vi "Configure Signal Track Enabled.vi"(8 "error in (no error)":errorcluster {"code" format="%.0x"}, 9 "signal track enabled (Off)":bool, 11 "instrument handle":refnum<k15>) -> (0 "error out":errorcluster {"code" format="%.0x"}, 3 "instrument handle out":refnum<k15>)   [LabVIEW 2009, in "Keysight XSAn.lvlib"]
doc: "This VI enables or disables signal-tracking.\n\nSupported Models: M9290A, N8973B, N8974B, N8975B, N8976B, N9000A, N9000B, N9010A, N9010B, N9020A, N9020B, N9030A, N9030B, N9038A, N9040B, N9041B, SPN9003A, SPN9026A"
uses:
  <instrlib>/Keysight XSAn/Keysight XSAn.lvlib
  AgXSAn.dll
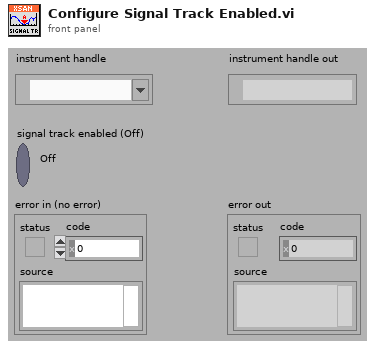
[diagram p1: front panel]
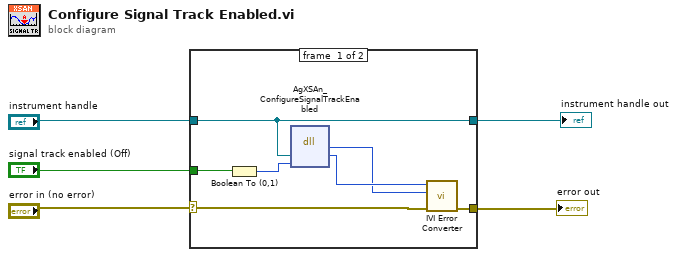
[diagram p0: block diagram]
diagram:
  n1 = case shown="No Error" "error in (no error)" {
    selector: "error in (no error)" -> [w9 w14]
    tunnel: [w10 w14] -> w4
    tunnel: "instrument handle" -> [w7 w13]
    tunnel: [w7 w13] -> w2
    tunnel: "signal track enabled (Off)" -> [w6 _]
    frame #0 {
      n2 = Boolean To (0,1)(Boolean=w6) -> (0, 1=w12:i16)
      n3 = dll-call lib="AgXSAn**.dll" fn="AgXSAn_ConfigureSignalTrackEnabled" ("LabVIEW:IviSpecAn_ConfigureSignalTrackEnabled")("instrument handle"=w7, "signal track enabled"=w12) -> ("Status"=w8:i32, "instrument handle"=w11:u32)  [unwired: 4 in, 2 out]
      n4 = call <instrlib>:"IVI Error Converter.vi"("error in (no error)"=w9, "IVI error code (0)"=w8, "instrument handle"=w11) -> ("error out"=w10:errorcluster)  [unwired: 7 in, 1 out]
    }
    frame #1 {
    }
  }
  "error out" <- w4
  "instrument handle out" <- w2
